vi "GEA2 Serial Send Index Error.vi"(8 "error in (no error)":errorcluster, 11 "Com Port":u8) -> (0 "error out":errorcluster)   [LabVIEW 2014]
uses:
  Type Definitions/GEA2 Serial Dryer Interface Ctrl.ctl
  Type Definitions/GEA2 Serial Dryer Commands.ctl
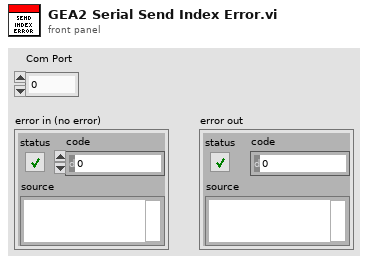
[diagram p1: front panel]
types:
  T1 = typedef "GEA2 Serial Dryer Commands.ctl" = u8
  T2 = typedef "GEA2 Serial Dryer Interface Ctrl.ctl" = enum16{"Init Com Port", "SendCMD", "ReadPort", "Close Port", "Simulate Diag Data", "Send WILT Startup CMDs", "Send Continue CMD", "Read Continuous"}
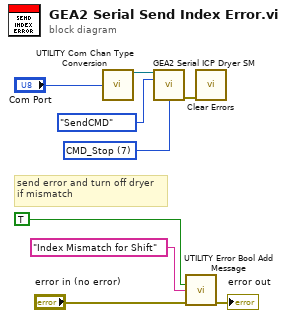
[diagram p0: block diagram]
diagram:
  w6 = T1 7 items=["CMD_Eval_Mode_Entry_CC1", "CMD_Eval_Mode_Entry_CC2", "CMD_Eval_Mode_Continue", "CMD_Send_DIAG_Info", "CMD_Enable_Debug_Log ", "CMD_Disable_Debug_Log ", "CMD_Send_Log_Data", "CMD_Stop", "RQST_Version"] ("Command")
  # "send error and turn off dryer\nif mismatch"
  n1 = call "UTILITY Com Chan Type Conversion.vi"("Com Chan"="Com Port") -> ("VISA resource name"=w7:refnum<visa-resource-name>)  [unwired: 11 in, 3 out]
  n2 = call "GEA2 Serial ICP Dryer SM.vi"("ComPort"=w7, "Mode"=GEA2_Serial_Dryer_Interface_Ctrl."SendCMD", "Command"=w6) -> ("Error Out"=w9:errorcluster)  [unwired: 8 in, 4 out]
  n3 = call "UTILITY Error Bool Add Message.vi"("Error?"=TRUE, "Message"="Index Mismatch for Shift", "Error In"="error in (no error)") -> ("Error Out"=→"error out":errorcluster)  [unwired: 12 in]
  n4 = call <vilib>:"Clear Errors.vi"("error in (no error)"=w9) -> ()  [unwired: 5 in, 2 out]
